vi "Keyboard Filter Master.vi"(0 "error in (no error)":errorcluster, 1 "install / remove filter":enum16{"Install Filter", "Remove Filter"}(ring)=enum."Remove Filter", 5 "filter types":T1) -> (3 "error out":errorcluster)   [LabVIEW 2020, in "MacroAssert.lvlib" / "WINKEY.lvlib"]
doc: "This VI allows you to install or remove a system-wide keyboard filter. The user can choose to disable the hot-key to show the Windows Task List (as well as selecting Switch To... from the System menu) and / or the <Alt> key combinations that allow one to switch to another Windows application. Note that double-clicking on the desktop will still bring up the Task List.\n\nInstalling a filter with both filter types set to OFF will also remove the filter. If a filter is already installed, and the function is called again, the new filter replaces the current filter."
uses:
  WINKEY.lvlib
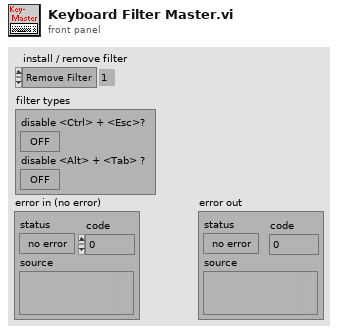
[diagram p1: front panel]
types:
  T1 = cluster{"disable <Ctrl> + <Esc>?":bool, "disable <Alt> + <Tab> ?":bool}
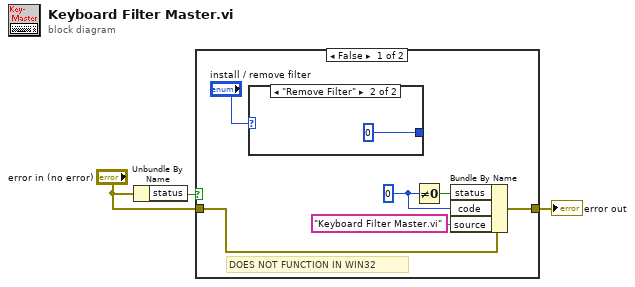
[diagram p0: block diagram]
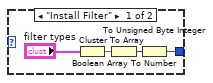
[diagram p2: hidden frame]
diagram:
  n1 = Unbundle By Name("error in (no error)") -> ("status"=w3:bool)
  n2 = case shown="False" w3 {
    tunnel: "error in (no error)" -> [w4 w15]
    tunnel: [w5 w15] -> w1
    frame False {
      w7 = 0 ("x")
      # "DOES NOT FUNCTION IN WIN32"
      n3 = case shown="\"Remove Filter\"" "install / remove filter" {
        tunnel: [w12 u8 0] -> _
        frame "Install Filter" {
          n4 = Cluster To Array(cluster="filter types") -> (array=w10:bool[])
          n5 = Boolean Array To Number(Boolean array=w10) -> (number=w13:u32)
          n6 = To Unsigned Byte Integer(number=w13) -> (unsigned 8bit integer=w12:u8)
        }
        frame "Remove Filter" {
        }
      }
      n7 = Not Equal To 0?(x=w7) -> (x != 0?=w8:bool)
      n8 = Bundle By Name(cluster=w4, "status"=w8, "code"=w7, "source"="Keyboard Filter Master.vi") -> (w5:errorcluster)
    }
    frame True {
    }
  }
  "error out" <- w1
